vi "SDP810-string-array-to-data.vi"(9 "Starting Index":i32, 11 "Data In (string array)":string[](array[string])) -> (0 "SDP810: data output":T1 {"Humidity (%)" format="%.2f"; "Temp (degC)" format="%.2f"}, 2 "SDP810: Temp (degC)":dbl format="%.2f", 3 "SDP810: diff Pressure (mBar)":dbl format="%.2f")   [LabVIEW 2021]
uses:
  SHT41.ctl
  SDP810.ctl
panel:
  out "SDP810: Temperature":string
  out "SDP810: diff Pressure":string
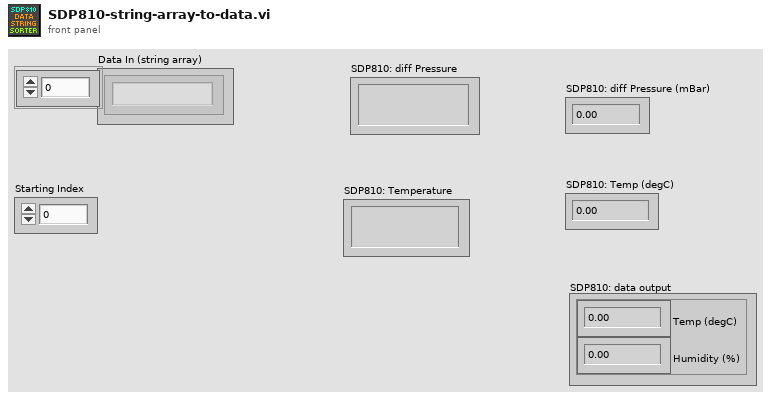
[diagram p1: front panel]
types:
  T1 = typedef "SHT41.ctl" = cluster{"Temp (degC)":dbl, "Humidity (%)":dbl}
  T2 = typedef "SDP810.ctl" = cluster{"dP (mBar)":dbl, "Temp (degC)":dbl}
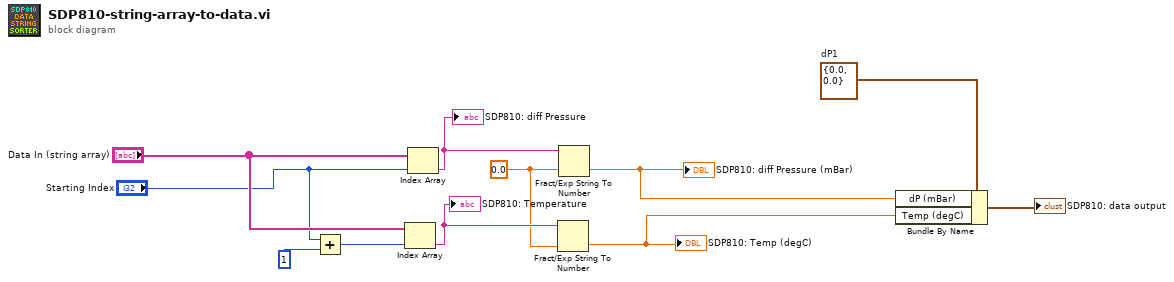
[diagram p0: block diagram]
diagram:
  w2 = T2 {"dP (mBar)"=0.0, "Temp (degC)"=0.0}  # dP1
  w5 = 0.0
  n1 = Add(x="Starting Index", y=1) -> (x+y=w9:i32)
  n2 = Index Array(array="Data In (string array)", index=w9) -> (element=w6:string)
  "SDP810: Temperature" <- w6
  n3 = Index Array "Index Array"(array="Data In (string array)", index="Starting Index") -> (element=w7:string)
  "SDP810: diff Pressure" <- w7
  n4 = Fract/Exp String To Number(string=w6, default (0 dbl)=w5) -> (number=w3:dbl)  [unwired: 2 in, 1 out]
  "SDP810: Temp (degC)" <- w3
  n5 = Fract/Exp String To Number(string=w7, default (0 dbl)=w5) -> (number=w4:dbl)  [unwired: 2 in, 1 out]
  "SDP810: diff Pressure (mBar)" <- w4
  n6 = Bundle By Name(cluster=w2, "dP (mBar)"=w4, "Temp (degC)"=w3) -> (→"SDP810: data output":T2)
